vi "cv1 max.vi"() -> ()   [LabVIEW 2023]
uses:
  <vilib>/DAQmx/write.llb/DAQmx Write (Analog Wfm 1Chan NSamp).vi
  <vilib>/DAQmx/read.llb/DAQmx Read (Analog Wfm 1Chan NSamp).vi
  <vilib>/DAQmx/create/channels.llb/DAQmx Create Channel (AI-Voltage-Basic).vi
  <vilib>/DAQmx/configure/timing.llb/DAQmx Timing (Sample Clock).vi
  <vilib>/DAQmx/miscellaneous.llb/DAQmx Fill In Error Info.vi
  <vilib>/DAQmx/create/channels.llb/DAQmx Create Channel (AO-Voltage-Basic).vi
  <vilib>/measure/NI_MABase.lvlib
panel:
  in  "stop 2":bool
  out "Waveform Graph 2":waveform(dbl)(graph)
  in  "stop":bool
  out "Waveform Graph":waveform(dbl)(graph)
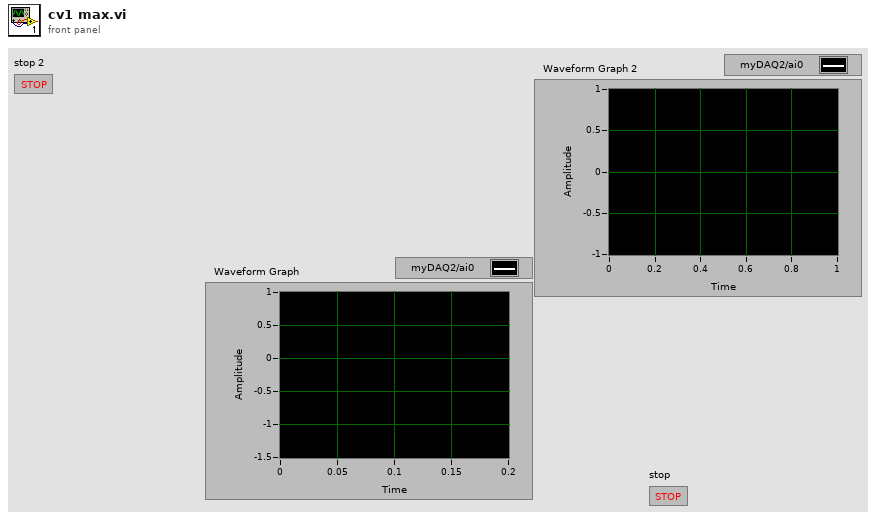
[diagram p1: front panel]
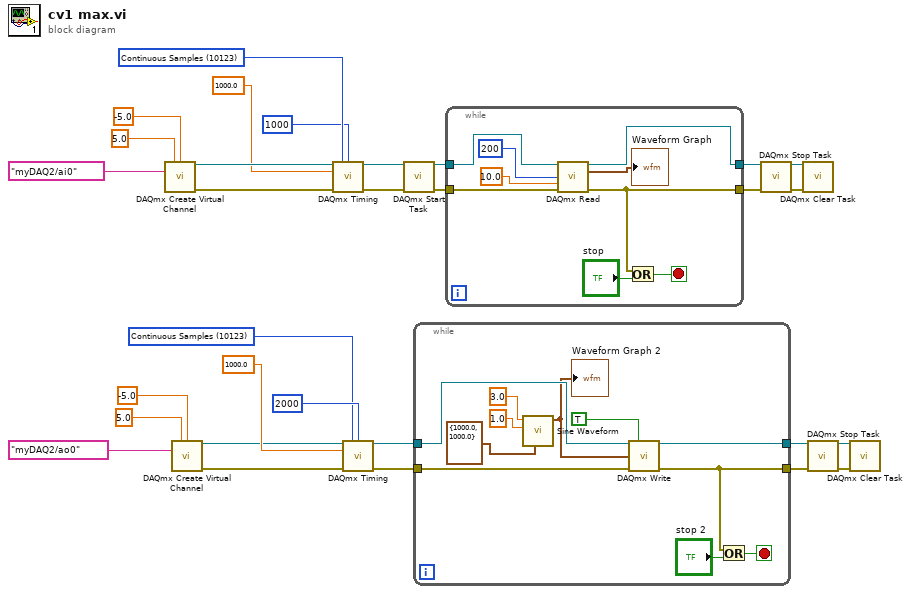
[diagram p0: block diagram]
diagram:
  w11 = 10123 items=["Finite Samples"=10178, "Continuous Samples"=10123, "Hardware Timed Single Point"=12522] ("sample mode")
  w24 = 10123 items=["Finite Samples"=10178, "Continuous Samples"=10123, "Hardware Timed Single Point"=12522] ("sample mode")
  n1 = call-poly <vilib>:"DAQmx Create Virtual Channel.vi"("maximum value"=5.0, "minimum value"=-5.0, "physical channels"=tag "myDAQ2/ai0") -> ("task out"=w27:refnum<k21>, "error out"=w26:errorcluster)  [unwired: 11 in]
  n2 = call-poly <vilib>:"DAQmx Create Virtual Channel.vi"("maximum value"=5.0, "minimum value"=-5.0, "physical channels"=tag "myDAQ2/ao0") -> ("task out"=w10:refnum<k21>, "error out"=w9:errorcluster)  [unwired: 11 in]
  n3 = call-poly <vilib>:"DAQmx Timing.vi"("task/channels in"=w27, "sample mode"=w24, "samples per channel"=1000, "rate"=1000.0, "error in"=w26) -> ("task out"=w22:refnum<k21>, "error out"=w21:errorcluster)  [unwired: 9 in]
  n4 = call-poly <vilib>:"DAQmx Timing.vi"("task/channels in"=w10, "sample mode"=w11, "samples per channel"=2000, "rate"=1000.0, "error in"=w9) -> ("task out"=w2:refnum<k21>, "error out"=w1:errorcluster)  [unwired: 9 in]
  n5 = call <vilib>:"DAQmx Start Task.vi"("task/channels in"=w22, "error in"=w21) -> ("task out"=w20:refnum<k21>, "error out"=w19:errorcluster)  [unwired: 12 in]
  n6 = while {
    tunnel: [w40] -> w4
    tunnel: [w32] -> w3
    tunnel: w2 -> [w39]
    tunnel: w1 -> [w38]
    stop <- w31 stop-if-true
    n7 = call <vilib>:"Sine Waveform.vi"("sampling info"=cluster{"Fs":dbl, "#s":dbl} {"Fs"=1000.0, "#s"=1000.0}, "amplitude"=1.0, "frequency"=3.0) -> ("signal out"=w34:waveform(dbl))  [unwired: 7 in, 1 out]
    "Waveform Graph 2" <- w34
    n8 = call-poly <vilib>:"DAQmx Write.vi"("task/channels in"=w39, "auto start"=TRUE, "data"=w34, "error in"=w38) -> ("task out"=w40:refnum<k21>, "error out"=w32:errorcluster)  [unwired: 9 in, 1 out]
    n9 = Or(x=w32, y="stop 2") -> (x .or. y?=w31:bool)
  }
  n10 = while {
    tunnel: w20 -> [w50]
    tunnel: w19 -> [w49]
    tunnel: [w45] -> w18
    tunnel: [w42] -> w17
    stop <- w43 stop-if-true
    n11 = call-poly <vilib>:"DAQmx Read.vi"("task/channels in"=w50, "number of samples per channel"=200, "timeout"=10.0, "error in"=w49) -> ("task out"=w45:refnum<k21>, "data"=→"Waveform Graph":waveform(dbl), "error out"=w42:errorcluster)  [unwired: 9 in]
    n12 = Or(x=w42, y="stop") -> (x .or. y?=w43:bool)
  }
  n13 = call <vilib>:"DAQmx Stop Task.vi"("task/channels in"=w18, "error in"=w17) -> ("task out"=w16:refnum<k21>, "error out"=w15:errorcluster)  [unwired: 12 in]
  n14 = call <vilib>:"DAQmx Clear Task.vi"("task in"=w16, "error in"=w15) -> ()  [unwired: 13 in, 1 out]
  n15 = call <vilib>:"DAQmx Stop Task.vi"("task/channels in"=w4, "error in"=w3) -> ("task out"=w6:refnum<k21>, "error out"=w5:errorcluster)  [unwired: 12 in]
  n16 = call <vilib>:"DAQmx Clear Task.vi"("task in"=w6, "error in"=w5) -> ()  [unwired: 13 in, 1 out]
